vi "Write Field.vi"(9 "Field":T1, 11 "CItemMatch in":refnum<class "CItemMatch.lvclass">) -> (3 "CItemMatch out":refnum<class "CItemMatch.lvclass">)   [LabVIEW 2020, in "DependencyInspection.lvlib" / "CItemMatch.lvclass"]
uses:
  CItemMatch.lvclass
  TypeDefs/Field.ctl
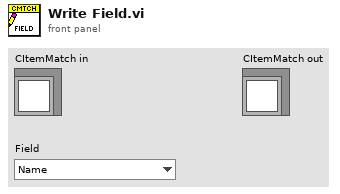
[diagram p1: front panel]
types:
  T1 = typedef "DependencyInspection.lvlib/CItemMatch.lvclass/Field.ctl" = enum16{"Name", "Qualified name", "Path"}
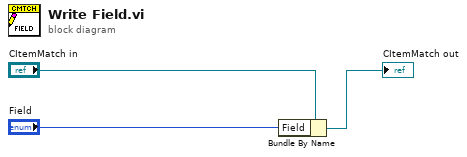
[diagram p0: block diagram]
diagram:
  n1 = Bundle By Name(cluster="CItemMatch in", "Field"="Field") -> (→"CItemMatch out":refnum<class "CItemMatch.lvclass">)
